vi "AKIP_read_voltage_current.vi"(8 "error in (no error)":errorcluster, 11 "VISA Refnum in":refnum<visa-resource-name>="AKIP") -> (0 "error out":errorcluster, 1 "Current":dbl, 2 "Voltage":dbl, 3 "VISA Refnum out":refnum<visa-resource-name>)   [LabVIEW 2017]
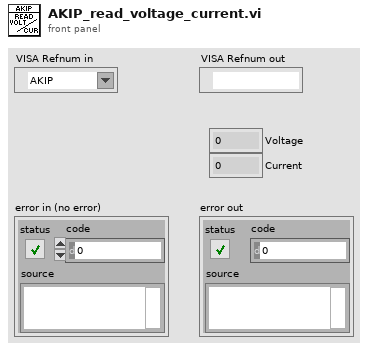
[diagram p1: front panel]
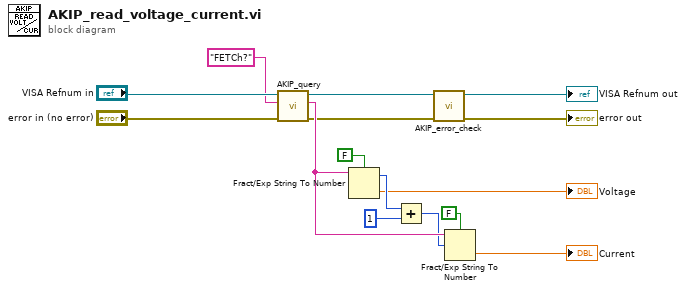
[diagram p0: block diagram]
diagram:
  n1 = call "AKIP_query.vi"("error in (no error)"="error in (no error)", "write buffer"="FETCh?", "VISA Refnum in"="VISA Refnum in") -> ("error out"=w5:errorcluster, "read buffer"=w15:string, "VISA Refnum out"=w6:refnum<visa-resource-name>)  [unwired: 6 in]
  n2 = Fract/Exp String To Number(use system decimal point (T)=FALSE, string=w15) -> (offset past number=w13:i32, number=→"Voltage":dbl)  [unwired: 2 in]
  n3 = Add(x=w13, y=1) -> (x+y=w12:i32)
  n4 = call "AKIP_error_check.vi"("error in (no error)"=w5, "VISA Refnum in"=w6) -> ("error out"=→"error out":errorcluster, "VISA Refnum out"=→"VISA Refnum out":refnum<visa-resource-name>)  [unwired: 8 in]
  n5 = Fract/Exp String To Number(use system decimal point (T)=FALSE, string=w15, offset=w12) -> (number=→"Current":dbl)  [unwired: 1 in, 1 out]
